vi "View.vi"() -> ()   [LabVIEW 2016]
uses:
  ElectrometerController/ElectrometerController.lvclass
  Test/Global 1.vi
  ElectrometerError/Controls/errorType.ctl
  ElectrometerError/ElectrometerError.lvclass
  Electrometer/State/ElectrometerState.lvclass
  Electrometer/Modes.ctl
  Electrometer/Electrometer.lvclass
panel:
  out "Reading":bool
  in  "Stop Reading":bool
  in  "Range":dbl=10.0
  in  "Duration":dbl
  in  "Intensity":dbl
  in  "Mode":T1
  in  "readUntilIntensity":bool
  out "Last Error":string
  out "Running":bool
  in  "Perform Zero Calib":bool
  in  "Change Measurement":bool
  in  "Start Read Set Duration":bool
  in  "Start Read Manual":bool
  out "error out":errorcluster
  in  "Stop":bool
  out "Measurement":dbl(graph)
  # "Controls"
  # "Status"
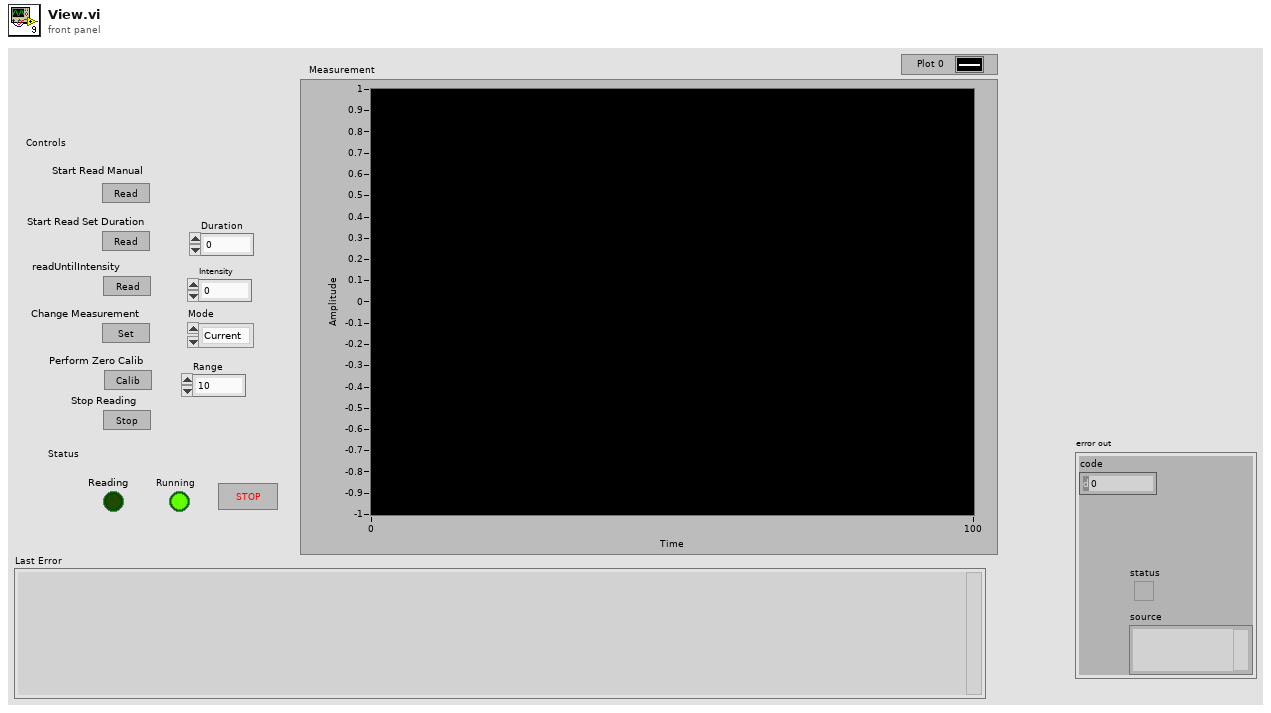
[diagram p1: front panel]
types:
  T1 = typedef "Electrometer.lvclass/Modes.ctl" = enum16{"Current", "Charge", "Voltage", "Resistance"}
  T2 = typedef "ElectrometerError.lvclass/errorType.ctl" = cluster{"errorType":enum16{"Error", "Warning", "None"}, "errorCode":dbl, "hwError":string, "salError":string}
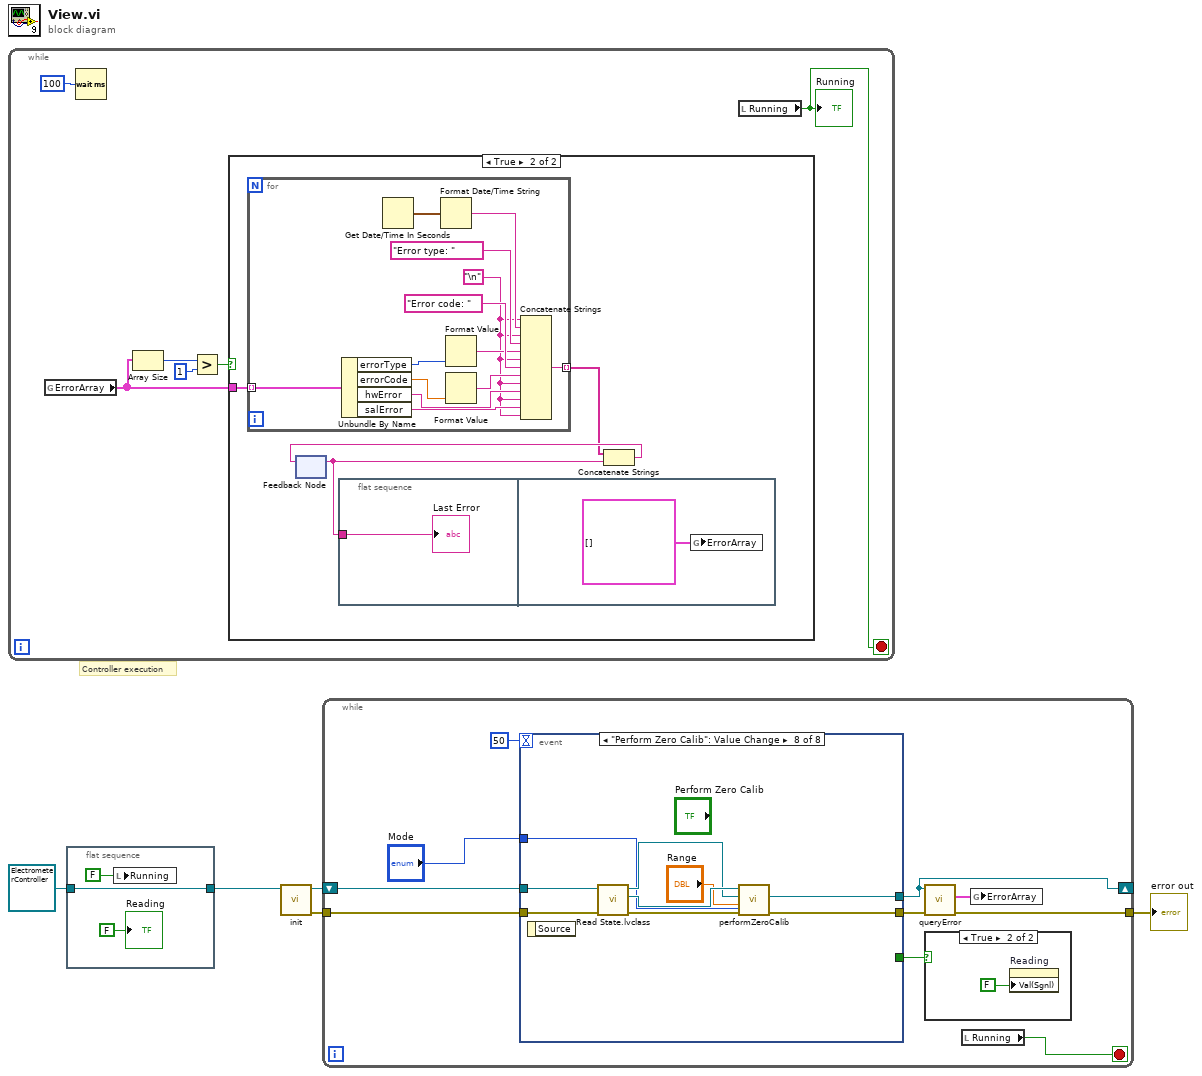
[diagram p0: block diagram]
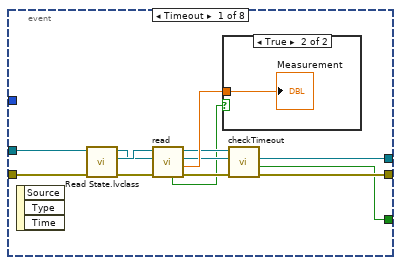
[diagram p3: hidden frame]
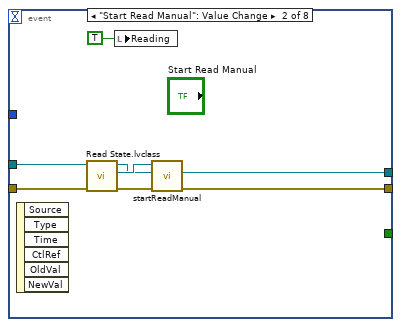
[diagram p5: hidden frame]
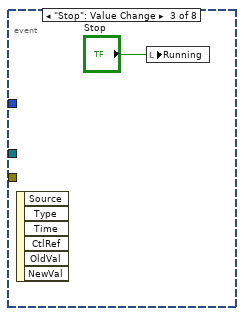
[diagram p6: hidden frame]
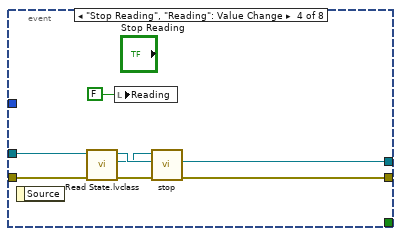
[diagram p7: hidden frame]
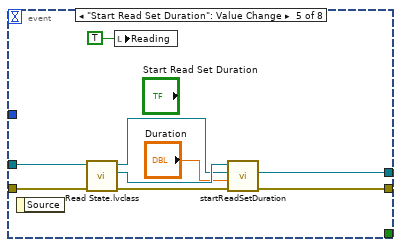
[diagram p8: hidden frame]
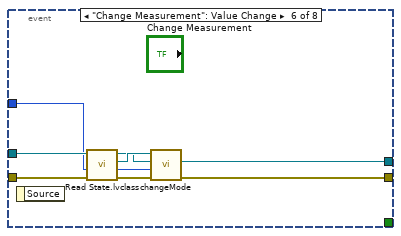
[diagram p9: hidden frame]
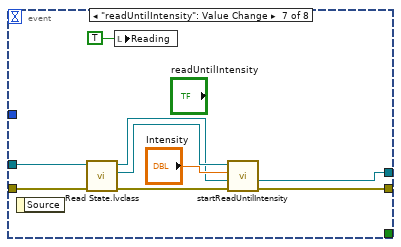
[diagram p10: hidden frame]
diagram:
  # "Controller execution"
  n1 = while {
    stop <- w10 stop-if-true
    n2 = global read "Global 1.vi" "ErrorArray"() -> (w9:T2[])
    n3 = Wait (ms)(milliseconds to wait=u32 100) -> ()  [unwired: 1 out]
    n4 = Array Size(array=w9) -> (size(s)=w7:i32)
    n5 = Greater?(x=w7, y=1) -> (0:w8:bool)
    n6 = case shown="True" w8 {
      tunnel: w9 -> [_ w15]
      frame False {
      }
      frame True {
        n7 = for {
          tunnel: w15 -> [w30] mode=indexing
          tunnel: [w29] -> w12 mode=indexing
          w18 = "\n"
          n8 = Unbundle By Name(w30) -> ("errorType"=w28:enum16{"Error", "Warning", "None"}, "errorCode"=w26:dbl, "hwError"=w23:string, "salError"=w24:string)
          n9 = Get Date/Time In Seconds() -> (seconds since 1Jan1904=w20:timestamp)
          n10 = Format Date/Time String(seconds (now)=w20) -> (date/time string=w19:string)  [unwired: 2 in]
          n11 = Format Value(value (0)=w28) -> (output string=w21:string)  [unwired: 2 in]
          n12 = Format Value(value (0)=w26) -> (output string=w25:string)  [unwired: 2 in]
          n13 = Concatenate Strings(w18, w19, w18, "Error type: ", w21, w18, "Error code: ", w25, w18, w23, w18, w24, w18) -> (w29:string)
        }
        n14 = feedback #1() -> (w13:string)  [unwired: 1 in]
        n15 = flat-sequence {
          tunnel: w13 -> [w16]
          frame #0 {
            "Last Error" <- w16
          }
          frame #1 {
            n16 = global write "Global 1.vi" "ErrorArray"(T2[] [] ("ErrorArray")) -> ()
          }
        }
        n17 = Concatenate Strings(w12, w13) -> (w14:string)
        n18 = feedback-in #1(w14) -> ()
      }
    }
    n19 = local read "Running"() -> (w10:bool)
    "Running" <- w10
  }
  n20 = flat-sequence {
    tunnel: refnum<class "ElectrometerController.lvclass"> refnum ("ElectrometerController.lvclass") -> [w33]
    tunnel: [w33] -> w4
    frame #0 {
      n21 = local write "Running"(FALSE ("Running")) -> ()
      "Reading" <- FALSE ("Reading")
    }
  }
  n22 = call-dynamic "init.vi"("ElectrometerController in"=w4) -> ("error out"=w3:errorcluster, "ElectrometerController out"=w1:refnum<class "ElectrometerController.lvclass">)  [unwired: 9 in]
  n23 = while {
    tunnel: w3 -> [w42]
    tunnel: [w34] -> w2
    shift-right: [w37] -> _
    shift-left: w1 -> [w38]
    stop <- w39 stop-if-true
    n24 = event shown="[7] \"Perform Zero Calib\": Value Change" {
      selector: _ -> [_ _ _ _ _ _ _ _]
      dyn-events: _ -> [_ _ _ _ _ _ _ _]
      timeout: 50 -> [_ _ _ _ _ _ _ _]
      tunnel: w38 -> [w56 w65 _ w75 w84 w92 w101 w109]
      tunnel: w42 -> [w57 w66 _ w74 w83 w91 w100 w110]
      tunnel: "Mode" -> [_ _ _ _ _ w90 _ w105]
      tunnel: [w48 w60 _ w70 w77 w85 w96 w102] -> w37
      tunnel: [w47 w61 _ w69 w78 w86 w97 w103] -> w35
      tunnel: [w46 _ _ _ _ _ _ _] -> w40
      event Timeout {
        n25 = event-data() -> ()  [unwired: 1 in, 3 out]
        n26 = call-dynamic "Read State.lvclass.vi"("error in (no error)"=w57, "ElectrometerController in"=w56) -> ("error out"=w53:errorcluster, "ElectrometerState"=w55:refnum<class "ElectrometerState.lvclass">, "ElectrometerController out"=w54:refnum<class "ElectrometerController.lvclass">)  [unwired: 7 in]
        n27 = call-dynamic "read.vi"("error in (no error)"=w53, "ElectrometerController in"=w54, "State in"=w55) -> ("error out"=w51:errorcluster, "lastMeasure"=w52:dbl, "ElectrometerController out"=w50:refnum<class "ElectrometerController.lvclass">, "State out"=w49:refnum<class "ElectrometerState.lvclass">, "newValue"=w45:bool)  [unwired: 4 in]
        n28 = case shown="True" w45 {
          tunnel: w52 -> [_ w58]
          frame False {
          }
          frame True {
            "Measurement" <- w58
          }
        }
        n29 = call-dynamic "checkTimeout.vi"("error in (no error)"=w51, "ElectrometerController in"=w50, "State in"=w49) -> ("error out"=w47:errorcluster, "timeout?"=w46:bool, "ElectrometerController out"=w48:refnum<class "ElectrometerController.lvclass">)  [unwired: 5 in, 1 out]
      }
      event "Start Read Manual": Value Change {
        n30 = event-data() -> ()  [unwired: 1 in, 6 out]
        n31 = call-dynamic "Read State.lvclass.vi"("error in (no error)"=w66, "ElectrometerController in"=w65) -> ("error out"=w64:errorcluster, "ElectrometerState"=w63:refnum<class "ElectrometerState.lvclass">, "ElectrometerController out"=w62:refnum<class "ElectrometerController.lvclass">)  [unwired: 7 in]
        n32 = local write "Reading"(TRUE ("Reading")) -> ()
        n33 = call-dynamic "startReadManual.vi"("error in (no error)"=w64, "ElectrometerController in"=w62, "State in"=w63) -> ("error out"=w61:errorcluster, "ElectrometerController. out"=w60:refnum<class "ElectrometerController.lvclass">)  [unwired: 6 in, 1 out]
      }
      event "Stop": Value Change {
        n34 = event-data() -> ()  [unwired: 1 in, 6 out]
        n35 = local write "Running"("Stop") -> ()
      }
      event "Stop Reading", "Reading": Value Change {
        n36 = event-data() -> ()  [unwired: 1 in, 1 out]
        n37 = call-dynamic "Read State.lvclass.vi"("error in (no error)"=w74, "ElectrometerController in"=w75) -> ("error out"=w71:errorcluster, "ElectrometerState"=w72:refnum<class "ElectrometerState.lvclass">, "ElectrometerController out"=w73:refnum<class "ElectrometerController.lvclass">)  [unwired: 7 in]
        n38 = local write "Reading"(FALSE ("Reading")) -> ()
        n39 = call-dynamic "stop.vi"("error in (no error)"=w71, "ElectrometerController int"=w73, "State in"=w72) -> ("error out"=w69:errorcluster, "ElectrometerController out"=w70:refnum<class "ElectrometerController.lvclass">)  [unwired: 6 in, 1 out]
      }
      event "Start Read Set Duration": Value Change {
        n40 = event-data() -> ()  [unwired: 1 in, 1 out]
        n41 = call-dynamic "Read State.lvclass.vi"("error in (no error)"=w83, "ElectrometerController in"=w84) -> ("error out"=w82:errorcluster, "ElectrometerState"=w81:refnum<class "ElectrometerState.lvclass">, "ElectrometerController out"=w80:refnum<class "ElectrometerController.lvclass">)  [unwired: 7 in]
        n42 = local write "Reading"(TRUE ("Reading")) -> ()
        n43 = call-dynamic "startReadSetDuration.vi"("error in (no error)"=w82, "duration"="Duration", "ElectrometerController in"=w80, "State in"=w81) -> ("error out"=w78:errorcluster, "ElectrometerController. out"=w77:refnum<class "ElectrometerController.lvclass">)  [unwired: 5 in, 1 out]
      }
      event "Change Measurement": Value Change {
        n44 = event-data() -> ()  [unwired: 1 in, 1 out]
        n45 = call-dynamic "Read State.lvclass.vi"("error in (no error)"=w91, "ElectrometerController in"=w92) -> ("error out"=w89:errorcluster, "ElectrometerState"=w88:refnum<class "ElectrometerState.lvclass">, "ElectrometerController out"=w87:refnum<class "ElectrometerController.lvclass">)  [unwired: 7 in]
        n46 = call-dynamic "changeMode.vi"("error in (no error)"=w89, 9:w90, "ElectrometerController in"=w87, "State in"=w88) -> ("error out"=w86:errorcluster, "ElectrometerController out"=w85:refnum<class "ElectrometerController.lvclass">)  [unwired: 5 in, 1 out]
      }
      event "readUntilIntensity": Value Change {
        n47 = event-data() -> ()  [unwired: 1 in, 1 out]
        n48 = call-dynamic "Read State.lvclass.vi"("error in (no error)"=w100, "ElectrometerController in"=w101) -> ("error out"=w98:errorcluster, "ElectrometerState"=w94:refnum<class "ElectrometerState.lvclass">, "ElectrometerController out"=w93:refnum<class "ElectrometerController.lvclass">)  [unwired: 7 in]
        n49 = local write "Reading"(TRUE ("Reading")) -> ()
        n50 = call-dynamic "startReadUntilIntensity.vi"("error in (no error)"=w98, "ElectrometerController in"=w93, "Intensity"="Intensity", "State in"=w94) -> ("error out"=w97:errorcluster, "ElectrometerController out"=w96:refnum<class "ElectrometerController.lvclass">)  [unwired: 5 in, 1 out]
      }
      event "Perform Zero Calib": Value Change {
        n51 = event-data() -> ()  [unwired: 1 in, 1 out]
        n52 = call-dynamic "Read State.lvclass.vi"("error in (no error)"=w110, "ElectrometerController in"=w109) -> ("error out"=w107:errorcluster, "ElectrometerState"=w108:refnum<class "ElectrometerState.lvclass">, "ElectrometerController out"=w106:refnum<class "ElectrometerController.lvclass">)  [unwired: 7 in]
        n53 = call-dynamic "performZeroCalib.vi"(6:w105, "error in (no error)"=w107, 9:"Range", "ElectrometerController in"=w106, "State in"=w108) -> ("error out"=w103:errorcluster, "ElectrometerController out"=w102:refnum<class "ElectrometerController.lvclass">)  [unwired: 3 in, 2 out]
      }
    }
    n54 = call-dynamic "queryError.vi"("error in (no error)"=w35, "ElectrometerController in"=w37) -> ("error out"=w34:errorcluster, "ErrorArray"=w36:T2[])  [unwired: 7 in, 1 out]
    n55 = case shown="True" w40 {
      frame False {
      }
      frame True {
        n56 = property on="Reading" class="Bool (strict)"("Val(Sgnl)"=FALSE ("Value (Signaling)")) -> ()  [unwired: 2 in, 2 out]
      }
    }
    n57 = local read "Running"() -> (w39:bool)
    n58 = global write "Global 1.vi" "ErrorArray"(w36) -> ()
  }
  "error out" <- w2
